vi "SwapInstanceVIUnusedName2 52.vi"(6 "Bindata & descr in":T1, 7 "type":u8, 8 "error in (no error)":errorcluster, 9 "dims":u8=3 min=1 max=3, 11 "kwarg_name":string="testarg") -> (0 "error out":errorcluster, 1 "Array 3D":u8[][][](array[numeric]), 2 "Array 2D":u8[][](array[numeric]), 3 "Array 1D":u8[](array[numeric]), 4 "Bindata & descr out":T1, 5 "bindata":u8[](array[numeric]))   [LabVIEW 2018]
uses:
  Bindata&description.ctl
  Bindata description.ctl
  2657e102-909c-4968-9fe6-c24ad386b120.vi
  935a987e-412b-4b42-96f0-0a4911d68c07.vi
  eb7c1121-937a-47b5-958f-f0299c1709f3.vi
  722257cb-47b3-448d-b629-9e1c04b09561.vi
  935a987e-412b-4b42-96f0-0a4911d68c07.vi/68ab4c47-782a-4262-ad8c-9159585bd936.vi
  eb7c1121-937a-47b5-958f-f0299c1709f3.vi/a0871eda-38e7-4d16-a24f-287f60c031ae.vi
  722257cb-47b3-448d-b629-9e1c04b09561.vi/7638aed5-e0f8-42d5-adf2-f9ce836de844.vi
  935a987e-412b-4b42-96f0-0a4911d68c07.vi/68ab4c47-782a-4262-ad8c-9159585bd936.vi/170f2713-243c-461d-9741-397dde826de4.vi
  eb7c1121-937a-47b5-958f-f0299c1709f3.vi/a0871eda-38e7-4d16-a24f-287f60c031ae.vi/071e4d45-5228-4d83-a11d-03df0a3baf85.vi
  722257cb-47b3-448d-b629-9e1c04b09561.vi/7638aed5-e0f8-42d5-adf2-f9ce836de844.vi/9f5533d2-3c78-4331-a53c-a526cb605c84.vi
  935a987e-412b-4b42-96f0-0a4911d68c07.vi/68ab4c47-782a-4262-ad8c-9159585bd936.vi/170f2713-243c-461d-9741-397dde826de4.vi/c41b139d-7761-4f8b-9748-3004c5e886ce.vi
  eb7c1121-937a-47b5-958f-f0299c1709f3.vi/a0871eda-38e7-4d16-a24f-287f60c031ae.vi/071e4d45-5228-4d83-a11d-03df0a3baf85.vi/6d6bbafd-3428-49f0-a15c-17444baa7992.vi
  722257cb-47b3-448d-b629-9e1c04b09561.vi/7638aed5-e0f8-42d5-adf2-f9ce836de844.vi/9f5533d2-3c78-4331-a53c-a526cb605c84.vi/05f54bc2-8b67-42dc-920c-26575065327c.vi
  check ID validity.vi
  LV-Julia_ZMQ-Roundtrip_lib.lvlib
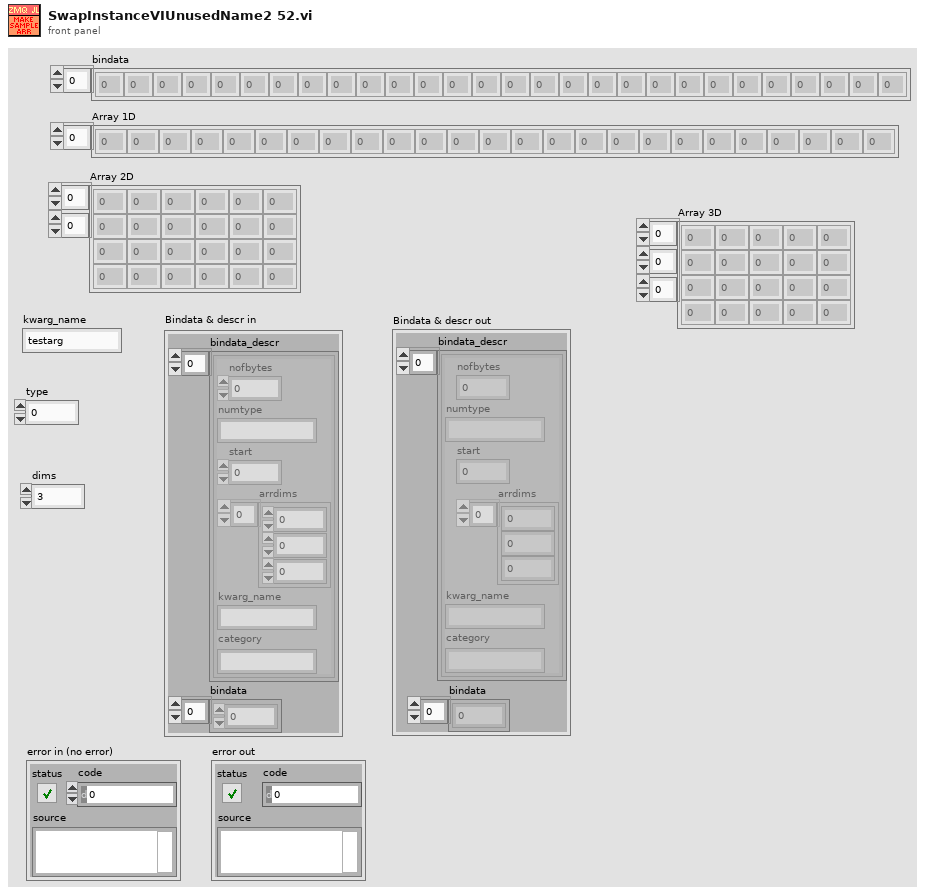
[diagram p1: front panel]
types:
  T1 = typedef "Bindata&description.ctl" = cluster{"bindata_descr":T2[], "bindata":u8[]}
  T2 = typedef "LV-Julia_ZMQ-Roundtrip_lib.lvlib/Bindata description.ctl" = cluster{"nofbytes":i32, "numtype":string, "start":i32, "arrdims":i32[], "kwarg_name":string, "category":string}
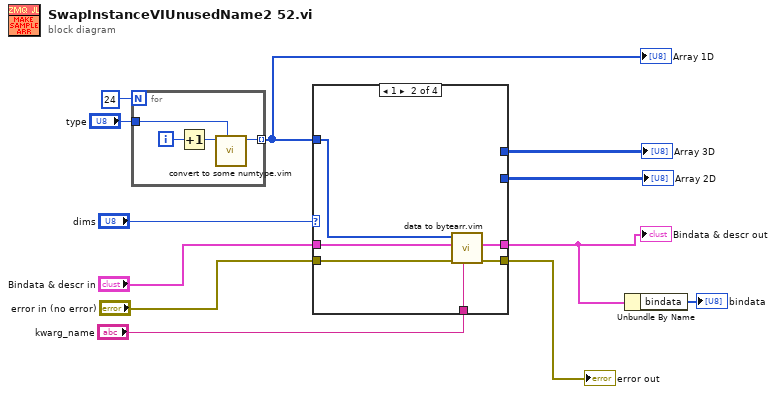
[diagram p0: block diagram]
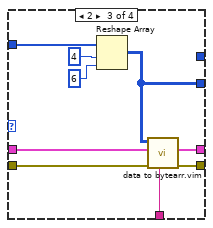
[diagram p3: hidden frame]
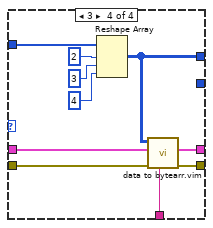
[diagram p4: hidden frame]
diagram:
  n1 = for {
    N: 24 -> [_]
    tunnel: [w14] -> w11 mode=indexing
    tunnel: "type" -> [w13]
    i -> [w16]
    n2 = Increment(x=w16) -> (x+1=w15:i32)
    n3 = call "convert to some numtype.vim"("type"=w13, "Numeric in"=w15) -> ("Numeric out"=w14:u8)  [unwired: 9 in]
  }
  "Array 1D" <- w11
  n4 = case shown="1" "dims" {
    tunnel: [_ _ _ w42] -> w12
    tunnel: w11 -> [_ w23 w30 w38]
    tunnel: "kwarg_name" -> [_ w22 w29 w37]
    tunnel: "error in (no error)" -> [w17 w21 w28 w36]
    tunnel: [w17 w20 w27 w35] -> w5
    tunnel: [_ w19 w26 w34] -> w2
    tunnel: [_ _ w25 _] -> w4
    tunnel: "Bindata & descr in" -> [_ w18 w24 w33]
    frame 0, Default {
    }
    frame 1 {
      n5 = call "data to bytearr.vim"("kwarg_name"=w22, "error in (no error)"=w21, "Bindata & descr in"=w18, "data in"=w23) -> ("error out"=w20:errorcluster, "Bindata & descr out"=w19:T1)  [unwired: 5 in, 1 out]
    }
    frame 2 {
      n6 = Reshape Array(w30, 4 ("dimension size"), 6 ("dimension size")) -> (w25:u8[][])
      n7 = call "data to bytearr.vim"("kwarg_name"=w29, "error in (no error)"=w28, "Bindata & descr in"=w24, "data in"=w25) -> ("error out"=w27:errorcluster, "Bindata & descr out"=w26:T1)  [unwired: 5 in, 1 out]
    }
    frame 3 {
      n8 = Reshape Array(w38, 2 ("dimension size"), 3 ("dimension size"), 4 ("dimension size")) -> (w42:u8[][][])
      n9 = call "data to bytearr.vim"("kwarg_name"=w37, "error in (no error)"=w36, "Bindata & descr in"=w33, "data in"=w42) -> ("error out"=w35:errorcluster, "Bindata & descr out"=w34:T1)  [unwired: 5 in, 1 out]
    }
  }
  "Array 3D" <- w12
  "Bindata & descr out" <- w2
  "error out" <- w5
  "Array 2D" <- w4
  n10 = Unbundle By Name(w2) -> ("bindata"=→"bindata":u8[])
